vi "WifiConnect.vi"(7 "连接延时":u32=2000, 8 "error in":errorcluster caption="错误输入（无错误）", 9 "cmd":string="baidu.com", 10 "Password":string="1234567890", 11 "WifiName":string="WIFI-180314-1454") -> (0 "error out":errorcluster caption="错误输出", 1 "Out":string, 2 "TimeSum":u32, 3 "Result？":bool)   [LabVIEW 2013]
panel:
  out "data out":string
  out "数据输出":string
  out "连接的字符串":string
  in  "连接后延时":u32=100
  in  "连接前延时":u32=100
  # "WIFI-180314-1454"
  # "Honor V10"
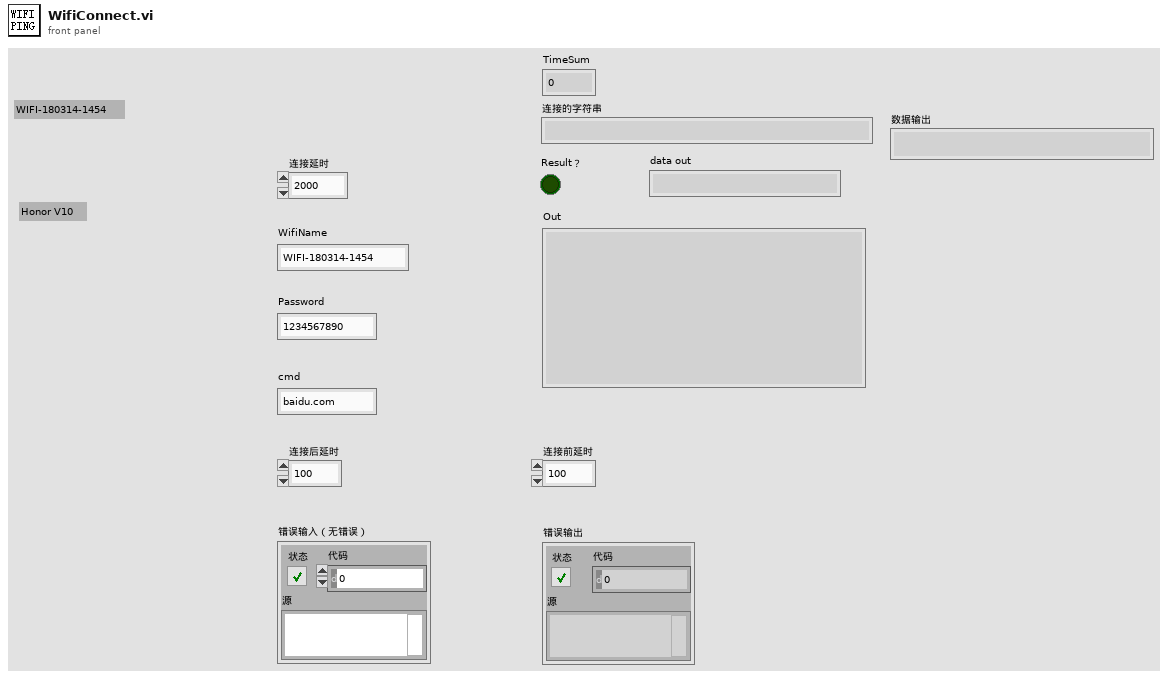
[diagram p1: front panel]
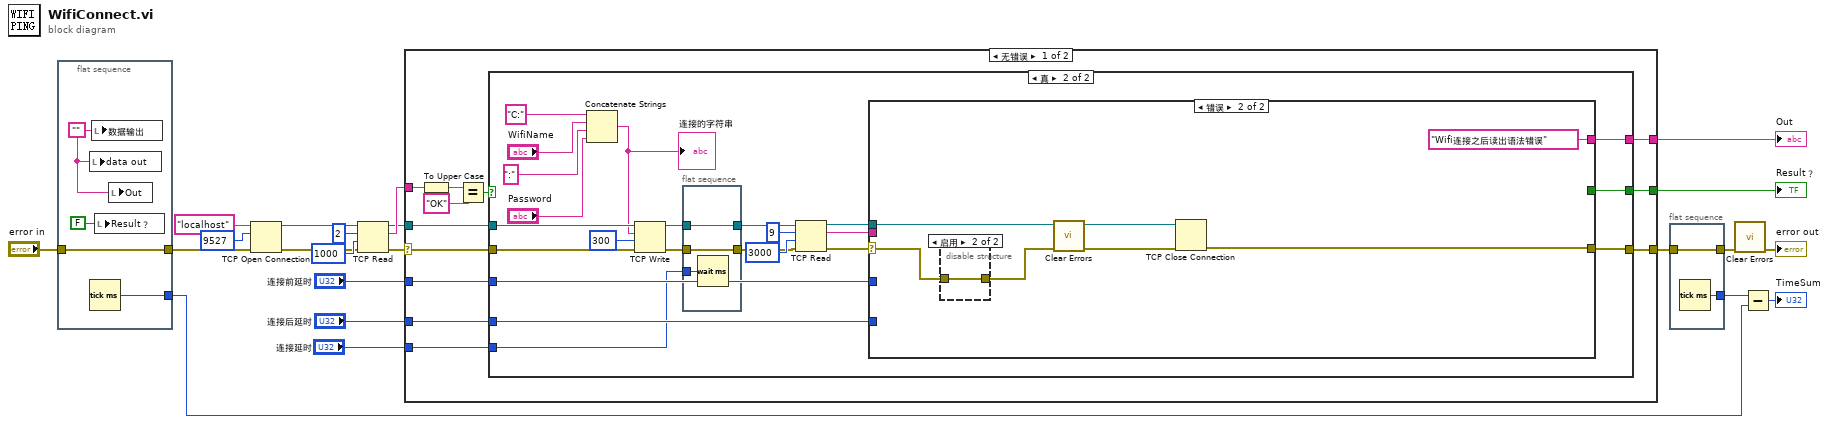
[diagram p0: block diagram]
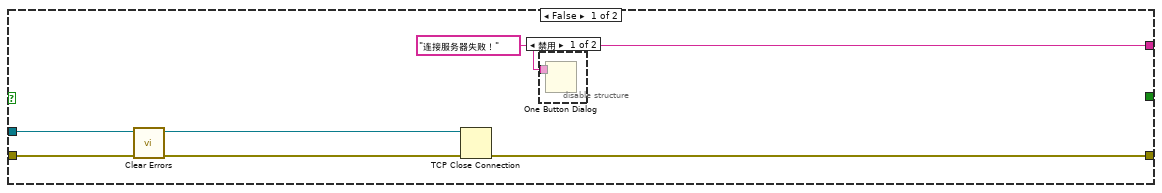
[diagram p2: hidden frame]
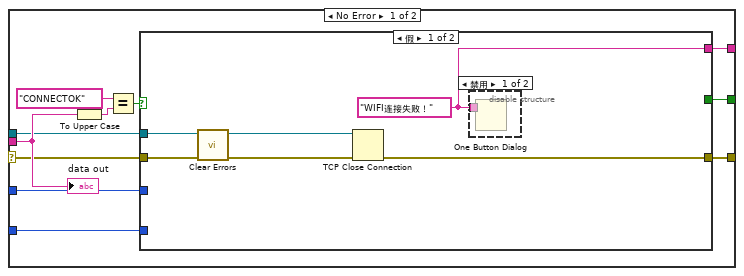
[diagram p4: hidden frame]
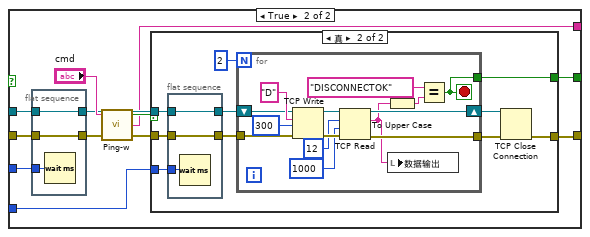
[diagram p6: hidden frame]
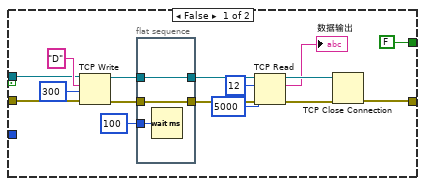
[diagram p7: hidden frame]
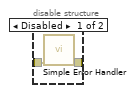
[diagram p8: hidden frame]
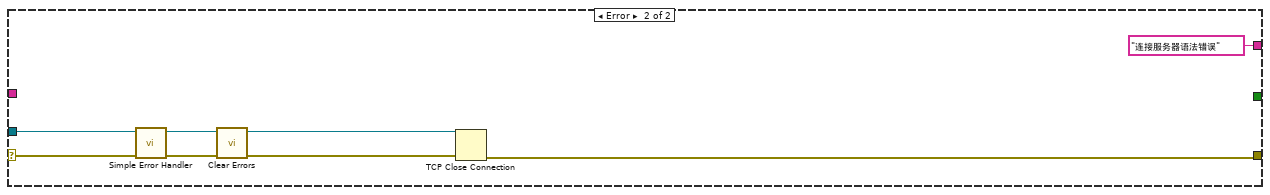
[diagram p9: hidden frame]
diagram:
  n1 = flat-sequence {
    tunnel: [w26] -> w8
    tunnel: "error in" -> [w26]
    tunnel: [w25] -> w3
    frame #0 {
      w24 = ""
      n2 = local write "data out"(w24) -> ()
      n3 = Tick Count (ms)() -> (millisecond timer value=w25:u32)
      n4 = local write "数据输出"(w24) -> ()
      n5 = local write "Result？"(FALSE ("Result？")) -> ()
      n6 = local write "Out"(w24) -> ()
    }
  }
  n7 = TCP Open Connection(address="localhost" ("名称"), remote port or service name=u16 9527 ("远程端口或服务名称"), error in (no error)=w8) -> (connection ID=w21:refnum<k5>, error out=w10:errorcluster)  [unwired: 2 in]
  n8 = TCP Read(connection ID=w21, bytes to read=2 ("读取的字节"), error in (no error)=w10, 9:1000 ("读取的字节")) -> (connection ID out=w16:refnum<k5>, data out=w18:string, error out=w17:errorcluster)  [unwired: 1 in]
  n9 = case shown="无错误" w17 {
    selector: w17 -> [w34 w163]
    tunnel: w18 -> [w38 _]
    tunnel: w16 -> [w33 w161]
    tunnel: "连接前延时" -> [w32 _]
    tunnel: "连接后延时" -> [w31 _]
    tunnel: [w30 w159] -> w6
    tunnel: [w29 "连接服务器语法错误" ("standard output")] -> w13
    tunnel: [w28 _] -> w12
    tunnel: "连接延时" -> [w27 _]
    frame No Error {
      n10 = To Upper Case(1:w38) -> (0:w37:string)
      n11 = Equal?(x=w37, y="OK" ("地址")) -> (x = y?=w35:bool)
      n12 = case shown="真" w35 {
        tunnel: w34 -> [w42 w66]
        tunnel: w33 -> [w43 w67]
        tunnel: w32 -> [_ w56]
        tunnel: w31 -> [_ w55]
        tunnel: [w40 w54] -> w30
        tunnel: [w39 w53] -> w29
        tunnel: [_ w52] -> w28
        tunnel: w27 -> [_ w49]
        frame False {
          w39 = "连接服务器失败！" ("消息")
          n13 = call <vilib>:"Clear Errors.vi"("error in (no error)"=w42) -> ("error out"=w41:errorcluster)  [unwired: 6 in]
          n14 = TCP Close Connection(connection ID=w43, error in (no error)=w41) -> (error out=w40:errorcluster)  [unwired: 1 in, 1 out]
          n15 = disable-structure shown="禁用" {
            disable-tunnel: w39 -> [w44 _]
            frame Disabled {
              n16 = One Button Dialog(message=w44) -> ()  [unwired: 1 in, 1 out]
            }
            frame Enabled {
            }
          }
        }
        frame True {
          n17 = Concatenate Strings("C:", "WifiName", ":", "Password") -> (w61:string)
          "连接的字符串" <- w61
          n18 = TCP Write(connection ID=w67, data in=w61, error in (no error)=w66, 9:300 ("读取的字节")) -> (connection ID out=w50:refnum<k5>, error out=w47:errorcluster)  [unwired: 1 out]
          n19 = flat-sequence {
            tunnel: [w70] -> w51
            tunnel: w50 -> [w70]
            tunnel: w49 -> [w69]
            tunnel: [w68] -> w48
            tunnel: w47 -> [w68]
            frame #0 {
              n20 = Wait (ms)(milliseconds to wait=w69) -> ()  [unwired: 1 out]
            }
          }
          n21 = TCP Read(connection ID=w51, bytes to read=9 ("读取的字节"), error in (no error)=w48, 9:3000 ("读取的字节")) -> (connection ID out=w57:refnum<k5>, data out=w46:string, error out=w45:errorcluster)  [unwired: 1 in]
          n22 = case shown="错误" w45 {
            selector: w45 -> [w77 w154]
            tunnel: w46 -> [w81 _]
            tunnel: w57 -> [w76 w153]
            tunnel: w56 -> [w75 _]
            tunnel: w55 -> [w74 _]
            tunnel: [w73 w150] -> w54
            tunnel: [w72 "Wifi连接之后读出语法错误" ("standard output")] -> w53
            tunnel: [w71 _] -> w52
            frame No Error {
              n23 = To Upper Case(1:w81) -> (0:w78:string)
              n24 = Equal?(x="CONNECTOK" ("地址"), y=w78) -> (x = y?=w80:bool)
              n25 = case shown="假" w80 {
                tunnel: w77 -> [w85 w96]
                tunnel: w76 -> [w86 w98]
                tunnel: w75 -> [_ w97]
                tunnel: w74 -> [_ w92]
                tunnel: [w83 w91] -> w73
                tunnel: [w82 w89] -> w72
                tunnel: [_ w88] -> w71
                frame False {
                  w82 = "WIFI连接失败！" ("消息")
                  n26 = call <vilib>:"Clear Errors.vi"("error in (no error)"=w85) -> ("error out"=w84:errorcluster)  [unwired: 6 in]
                  n27 = TCP Close Connection(connection ID=w86, error in (no error)=w84) -> (error out=w83:errorcluster)  [unwired: 1 in, 1 out]
                  n28 = disable-structure shown="禁用" {
                    disable-tunnel: w82 -> [w87 _]
                    frame Disabled {
                      n29 = One Button Dialog(message=w87) -> ()  [unwired: 1 in, 1 out]
                    }
                    frame Enabled {
                    }
                  }
                }
                frame True {
                  n30 = flat-sequence {
                    tunnel: w98 -> [w148]
                    tunnel: [w148] -> w94
                    tunnel: w97 -> [w147]
                    tunnel: w96 -> [w146]
                    tunnel: [w146] -> w95
                    frame #0 {
                      n31 = Wait (ms)(milliseconds to wait=w147) -> ()  [unwired: 1 out]
                    }
                  }
                  n32 = call "Ping-w.vi"("error in"=w95, "cmd"="cmd") -> ("error out"=w93:errorcluster, "standard output"=w89:string, "Acess"=w90:bool)  [unwired: 1 in]
                  n33 = case shown="真" w90 {
                    tunnel: w94 -> [w111 w128]
                    tunnel: w93 -> [w110 w125]
                    tunnel: w92 -> [_ w124]
                    tunnel: [w115 w122] -> w91
                    tunnel: [FALSE w119] -> w88
                    frame False {
                      n34 = TCP Write(connection ID=w111, data in="D", error in (no error)=w110, 9:300 ("读取的字节")) -> (connection ID out=w104:refnum<k5>, error out=w102:errorcluster)  [unwired: 1 out]
                      n35 = flat-sequence {
                        tunnel: [w118] -> w103
                        tunnel: w104 -> [w118]
                        tunnel: u32 100 ("连接延时") -> [w117]
                        tunnel: [w116] -> w101
                        tunnel: w102 -> [w116]
                        frame #0 {
                          n36 = Wait (ms)(milliseconds to wait=w117) -> ()  [unwired: 1 out]
                        }
                      }
                      n37 = TCP Read(connection ID=w103, bytes to read=12 ("读取的字节"), error in (no error)=w101, 9:5000 ("超时毫秒(25000)")) -> (connection ID out=w107:refnum<k5>, data out=→"数据输出":string, error out=w105:errorcluster)  [unwired: 1 in]
                      n38 = TCP Close Connection(connection ID=w107, error in (no error)=w105) -> (error out=w115:errorcluster)  [unwired: 1 in, 1 out]
                    }
                    frame True {
                      n39 = flat-sequence {
                        tunnel: w128 -> [w145]
                        tunnel: [w145] -> w127
                        tunnel: [w144] -> w126
                        tunnel: w125 -> [w144]
                        tunnel: w124 -> [w143]
                        frame #0 {
                          n40 = Wait (ms)(milliseconds to wait=w143) -> ()  [unwired: 1 out]
                        }
                      }
                      n41 = for {
                        N: 2 -> [_]
                        tunnel: w126 -> [w133]
                        tunnel: [w132] -> w123
                        shift-right: [w131] -> w121
                        shift-left: w127 -> [w134]
                        tunnel: [w130] -> w119
                        stop <- w130 stop-if-true
                        n42 = TCP Write(connection ID=w134, data in="D", error in (no error)=w133, 9:300 ("读取的字节")) -> (connection ID out=w139:refnum<k5>, error out=w140:errorcluster)  [unwired: 1 out]
                        n43 = TCP Read(connection ID=w139, bytes to read=12 ("读取的字节"), error in (no error)=w140, 9:1000 ("读取的字节")) -> (connection ID out=w131:refnum<k5>, data out=w129:string, error out=w132:errorcluster)  [unwired: 1 in]
                        n44 = To Upper Case(1:w129) -> (0:w138:string)
                        n45 = local write "数据输出"(w129) -> ()
                        n46 = Equal?(x="DISCONNECTOK" ("地址"), y=w138) -> (x = y?=w130:bool)
                      }
                      n47 = TCP Close Connection(connection ID=w121, error in (no error)=w123) -> (error out=w122:errorcluster)  [unwired: 1 in, 1 out]
                    }
                  }
                }
              }
              "data out" <- w81
            }
            frame Error {
              n48 = disable-structure shown="启用" {
                disable-tunnel: w154 -> [w156 w157]
                disable-tunnel: [w155 w157] -> w152
                frame Disabled {
                  n49 = call <vilib>:"Simple Error Handler.vi"("error in (no error)"=w156) -> ("error out"=w155:errorcluster)  [unwired: 4 in, 4 out]
                }
                frame Enabled {
                }
              }
              n50 = call <vilib>:"Clear Errors.vi"("error in (no error)"=w152) -> ("error out"=w151:errorcluster)  [unwired: 6 in]
              n51 = TCP Close Connection(connection ID=w153, error in (no error)=w151) -> (error out=w150:errorcluster)  [unwired: 1 in, 1 out]
            }
          }
        }
      }
    }
    frame Error {
      n52 = call <vilib>:"Simple Error Handler.vi"("error in (no error)"=w163) -> ("error out"=w162:errorcluster)  [unwired: 4 in, 4 out]
      n53 = call <vilib>:"Clear Errors.vi"("error in (no error)"=w162) -> ("error out"=w160:errorcluster)  [unwired: 6 in]
      n54 = TCP Close Connection(connection ID=w161, error in (no error)=w160) -> (error out=w159:errorcluster)  [unwired: 1 in, 1 out]
    }
  }
  "Result？" <- w12
  "Out" <- w13
  n55 = flat-sequence {
    tunnel: w6 -> [w165]
    tunnel: [w165] -> w5
    tunnel: [w164] -> w4
    frame #0 {
      n56 = Tick Count (ms)() -> (millisecond timer value=w164:u32)
    }
  }
  n57 = call <vilib>:"Clear Errors.vi"("error in (no error)"=w5) -> ("error out"=→"error out":errorcluster)  [unwired: 6 in]
  n58 = Subtract(x=w4, y=w3) -> (x-y=→"TimeSum":u32)
